vi "GetFilterList.vi"(4 "Error in":errorcluster, 6 "Write":bool, 7 "Filter names in":string[](array[string])) -> (0 "Error out":errorcluster, 3 "Filter names out":string[](array[string]))   [LabVIEW 2019]
doc: "Ce VI ouvre le fichier de sauvegarde des modèles et lit les positions du modèle spécifié."
uses:
  <vilib>/Utility/config.llb/Read Key (String).vi
  <vilib>/Utility/config.llb/Write Key (String).vi
  <vilib>/Utility/config.llb/NI_LVConfig.lvlib
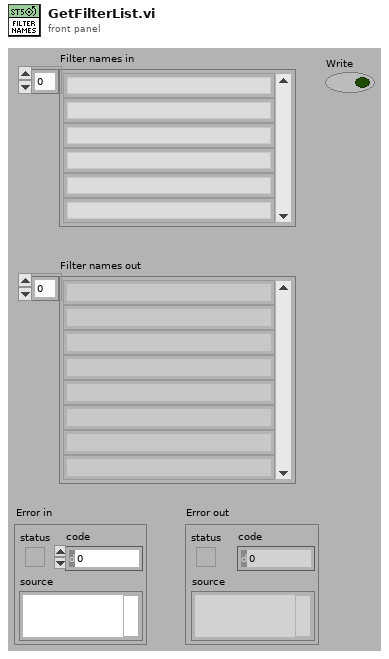
[diagram p1: front panel]
types:
  T1 = typedef "NI_LVConfig.lvlib/Config Data RefNum.ctl" = refnum<k1>
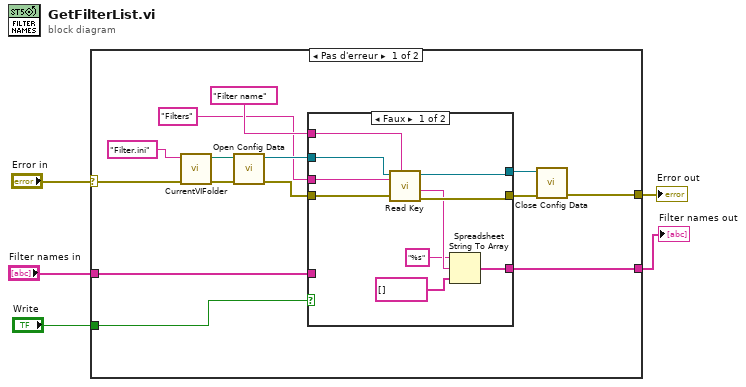
[diagram p0: block diagram]
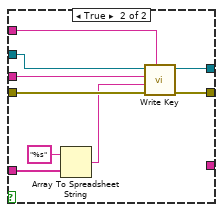
[diagram p2: hidden frame]
diagram:
  n1 = case shown="Pas d'erreur" "Error in" {
    selector: "Error in" -> [w13 w39]
    tunnel: [w12 w39] -> w5
    tunnel: "Filter names in" -> [w9 _]
    tunnel: "Write" -> [w8 _]
    tunnel: [w6 _] -> w1
    frame No Error {
      n2 = call <userlib>:"CurrentVIFolder.vi"("error in (no error)"=w13, "NomFichier"="Filter.ini") -> ("error out"=w19:errorcluster, "Chemin"=w11:path)  [unwired: 7 in, 1 out]
      n3 = call <vilib>:"Open Config Data.vi"("error in (no error)"=w19, "configuration file path"=w11) -> ("error out"=w15:errorcluster, "refnum"=w18:T1)  [unwired: 7 in, 1 out]
      n4 = case shown="Faux" w8 {
        tunnel: w18 -> [w26 w31]
        tunnel: "Filter name" ("section") -> [w28 w38]
        tunnel: [w25 w37] -> w16
        tunnel: w15 -> [w29 w36]
        tunnel: [w24 w35] -> w14
        tunnel: w9 -> [_ w32]
        tunnel: "Filters" ("section") -> [w27 w30]
        tunnel: [w20 _] -> w6
        frame False {
          n5 = call-poly <vilib>:"Read Key.vi"("section"=w28, "error in (no error)"=w29, "key"=w27, "refnum"=w26) -> ("error out"=w24:errorcluster, "value"=w23:string, "refnum out"=w25:T1)  [unwired: 4 in, 1 out]
          n6 = Spreadsheet String To Array(format string="%s" ("chaîne de format"), spreadsheet string=w23, array type (2D Dbl)=string[] [] ("Filter names in")) -> (array=w20:string[])  [unwired: 1 in]
        }
        frame True {
          n7 = Array To Spreadsheet String(array=w32, 3:"%s" ("chaîne de format")) -> (spreadsheet string=w33:string)  [unwired: 1 in]
          n8 = call-poly <vilib>:"Write Key.vi"("section"=w38, "error in (no error)"=w36, "value"=w33, "key"=w30, "refnum"=w31) -> ("error out"=w35:errorcluster, "refnum out"=w37:T1)  [unwired: 4 in, 1 out]
        }
      }
      n9 = call <vilib>:"Close Config Data.vi"("error in (no error)"=w14, "refnum"=w16) -> ("error out"=w12:errorcluster)  [unwired: 8 in, 1 out]
    }
    frame Error {
    }
  }
  "Error out" <- w5
  "Filter names out" <- w1
